vi "Windows Reboot.vi"() -> ()   [LabVIEW 2012]
uses:
  Windows/System32/user32.dll
panel:
  out "error out":errorcluster
  out "Boolean array":bool[](array[boolean])
  out "x .and. y?":u32
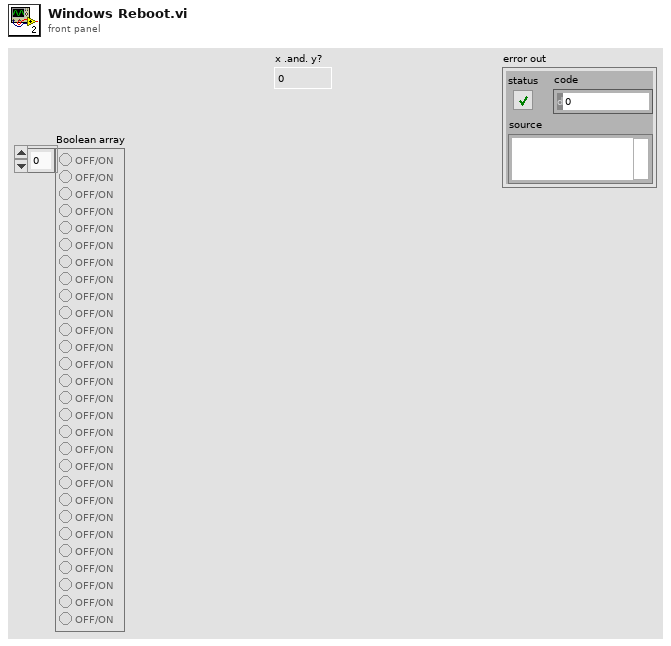
[diagram p1: front panel]
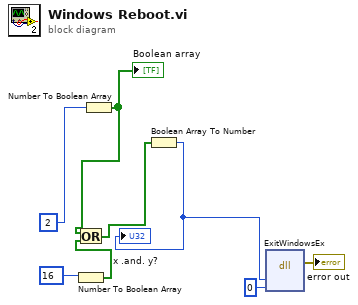
[diagram p0: block diagram]
diagram:
  n1 = Number To Boolean Array(number=u32 16) -> (Boolean array=w7:bool[])
  n2 = Number To Boolean Array(number=u32 2) -> (Boolean array=w6:bool[])
  "Boolean array" <- w6
  n3 = Or(x=w6, y=w7) -> (x .or. y?=w5:bool[])
  n4 = Boolean Array To Number(Boolean array=w5) -> (number=w1:u32)
  "x .and. y?" <- w1
  n5 = dll-call lib="C:/Windows/System32/user32.dll" fn="ExitWindowsEx"("uFlags"=w1, "dwReason"=u32 0) -> (error out=→"error out":errorcluster)  [unwired: 6 in, 1 out]
